vi "DivideToByte.vi"(2 "Offset":dbl format="%#_16g", 3 "Resolution":dbl format="%#_16g", 4 "Value":dbl format="%#_16g") -> (0 "HighByte":u8, 1 "LowByte":u8)   [LabVIEW 2013]
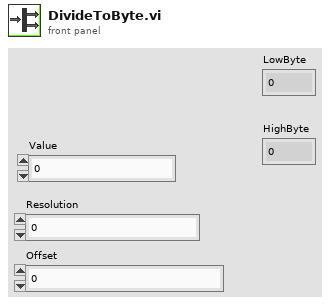
[diagram p1: front panel]
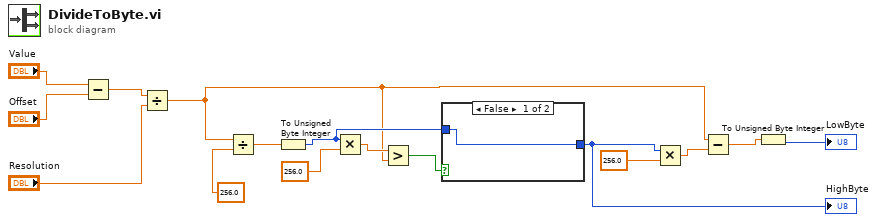
[diagram p0: block diagram]
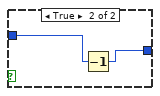
[diagram p2: hidden frame]
diagram:
  n1 = Subtract(x="Value", y="Offset") -> (x-y=w1:dbl)
  n2 = Divide(x=w1, y="Resolution") -> (x/y=w5:dbl)
  n3 = Divide(x=w5, y=256.0) -> (x/y=w12:dbl)
  n4 = To Unsigned Byte Integer(number=w12) -> (unsigned 8bit integer=w8:u8)
  n5 = Multiply(x=w8, y=256.0) -> (x*y=w10:dbl)
  n6 = Greater?(x=w10, y=w5) -> (0:w9:bool)
  n7 = case shown="False" w9 {
    tunnel: w8 -> [w17 w19]
    tunnel: [w17 w18] -> w2
    frame False {
    }
    frame True {
      n8 = Decrement(x=w19) -> (x-1=w18:u8)
    }
  }
  "HighByte" <- w2
  n9 = Multiply(x=w2, y=256.0) -> (x*y=w6:dbl)
  n10 = Subtract(x=w5, y=w6) -> (x-y=w4:dbl)
  n11 = To Unsigned Byte Integer(number=w4) -> (unsigned 8bit integer=→"LowByte":u8)
